vi "Remove non alphanum chars.vi"(8 "error in (no error)":errorcluster, 9 "Keep inner spaces (n)?":bool, 10 "Capitalize (n)?":bool, 11 "String In":string) -> (0 "error out":errorcluster, 3 "String Out":string)   [LabVIEW 2013]
uses:
  <vilib>/Utility/error.llb/whitespace.ctl
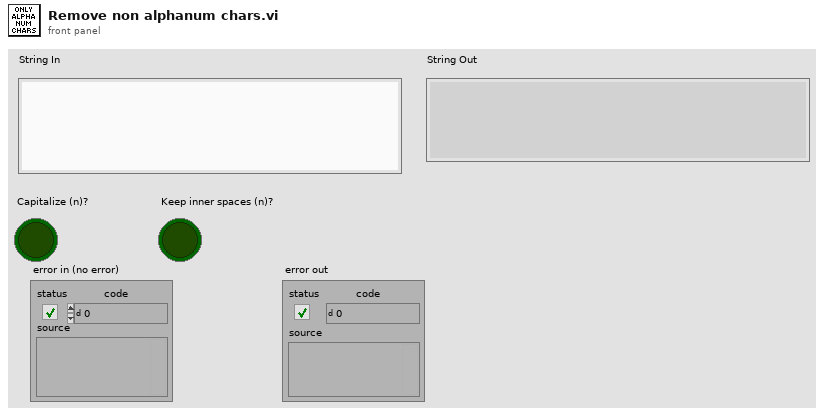
[diagram p1: front panel]
types:
  T1 = typedef "whitespace.ctl" = u16
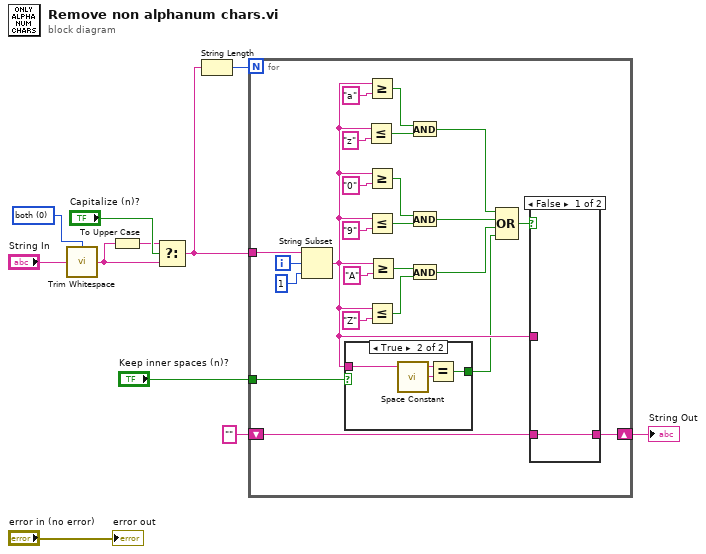
[diagram p0: block diagram]
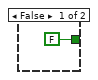
[diagram p2: hidden frame]
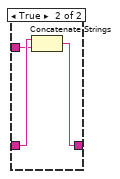
[diagram p3: hidden frame]
diagram:
  w11 = T1 0 items=["both", "start of string", "end of string"] ("location (both)")
  n1 = call <vilib>:"Trim Whitespace.vi"("string"="String In", "location (both)"=w11) -> ("trimmed string"=w2:string)
  n2 = To Upper Case(1:w2) -> (0:w5:string)
  n3 = Select(t=w5, s="Capitalize (n)?", f=w2) -> (s? t:f=w3:string)
  n4 = String Length(string=w3) -> (length=w10:i32)
  n5 = for {
    N: w10 -> [_]
    shift-right: [w15] -> w8
    shift-left: "" -> [w35]
    tunnel: w3 -> [w34]
    tunnel: "Keep inner spaces (n)?" -> [w14]
    i -> [w33]
    n6 = String Subset(string=w34, offset (0)=w33, length (rest)=1 ("length (rest)")) -> (substring=w13:string)
    n7 = case shown="True" w14 {
      tunnel: w13 -> [_ w39]
      tunnel: [FALSE w37] -> w12
      frame False {
      }
      frame True {
        n8 = call <vilib>:"Space Constant.vi"() -> ("String"=w38:string)
        n9 = Equal?(x=w39, y=w38) -> (x = y?=w37:bool)
      }
    }
    n10 = Less Or Equal?(x=w13, y="z") -> (x <= y?=w24:bool)
    n11 = Greater Or Equal?(x=w13, y="a") -> (x >= y?=w25:bool)
    n12 = Greater Or Equal?(x=w13, y="0") -> (x >= y?=w27:bool)
    n13 = Less Or Equal?(x=w13, y="9") -> (x <= y?=w26:bool)
    n14 = Less Or Equal?(x=w13, y="Z") -> (x <= y?=w23:bool)
    n15 = Greater Or Equal?(x=w13, y="A") -> (x >= y?=w22:bool)
    n16 = And(x=w25, y=w24) -> (x .and. y?=w19:bool)
    n17 = And(x=w27, y=w26) -> (x .and. y?=w18:bool)
    n18 = And(x=w22, y=w23) -> (x .and. y?=w17:bool)
    n19 = Compound Arithmetic op=OR(w19, w18, w17, w12) -> (w16:bool)
    n20 = case shown="False" w16 {
      tunnel: w35 -> [w40 w43]
      tunnel: w13 -> [_ w42]
      tunnel: [w40 w41] -> w15
      frame False {
      }
      frame True {
        n21 = Concatenate Strings(w43, w42) -> (w41:string)
      }
    }
  }
  "String Out" <- w8
  "error out" <- "error in (no error)"
